vi "Data Analog Output.vi"(0 "VISA resource name":refnum<visa-resource-name>, 7 "Analog Output (0: 1)":u16(ring) items=["1", "2"], 11 "error in (no error)":errorcluster) -> (4 "VISA resource name out":refnum<visa-resource-name>, 8 "Output Value":dbl min=-100.0 max=100.0 step=0.1 format="%.1f", 15 "error out":errorcluster)   [LabVIEW 2019, in "Lake Shore Cryotronics 340.lvlib"]
doc: "This VI querys the instrument for the percentage of output of an analog output."
uses:
  Lake Shore Cryotronics 340.lvlib
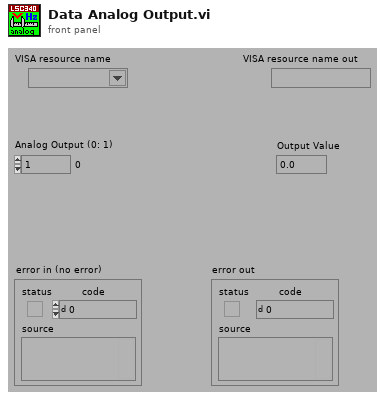
[diagram p1: front panel]
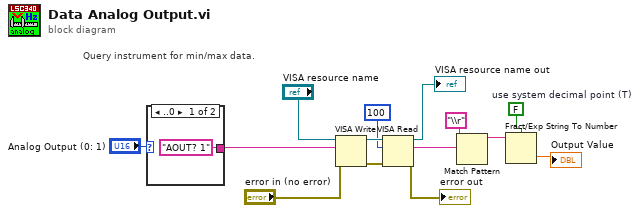
[diagram p0: block diagram]
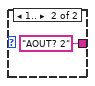
[diagram p2: hidden frame]
diagram:
  w1 = FALSE  # use system decimal point (T)
  # "Query instrument for min/max data."
  n1 = case shown="..0" "Analog Output (0: 1)" {
    tunnel: ["AOUT? 1" "AOUT? 2"] -> w2
    frame ..0 {
    }
    frame 1.. {
    }
  }
  n2 = VISA Write(VISA resource name="VISA resource name", write buffer=w2, error in (no error)="error in (no error)") -> (VISA resource name out=w12:refnum<visa-resource-name>, error out=w11:errorcluster)  [unwired: 1 out]
  n3 = VISA Read(VISA resource name=w12, byte count=100, error in (no error)=w11) -> (VISA resource name out=→"VISA resource name out":refnum<visa-resource-name>, read buffer=w9:string, error out=→"error out":errorcluster)  [unwired: 1 out]
  n4 = Match Pattern(string=w9, regular expression="\\r") -> (before substring=w7:string)  [unwired: 1 in, 3 out]
  n5 = Fract/Exp String To Number(use system decimal point (T)=w1, string=w7) -> (number=→"Output Value":dbl)  [unwired: 2 in, 1 out]
